vi "Localization.vi"(10 "parameter":string, 11 "Unlocalized":string="Launched") -> (3 "Localized":string="Launched TSS Server !")   [LabVIEW 2025, in "Config Tool.lvlib"]
doc: "This VI is used to provide localization -- that is, support for other human languages -- in the user interface. Given an input string, this VI returns the string that should be displayed for the current language. The idea is that you as a developer can use the Export/Import Strings feature of LabVIEW to produce a file that a translator can localize. The convention is that any control with \"DNL_\" as its label is skipped during localization (in English, this stands for Do Not Localize). The first array in this VI is one of these DNL_ controls. This array has the fixed strings that the program uses. The second array has the translated strings. Using this for all user visible text is sometimes cumbersome on the programmer, but it limits how many VIs have to be reviewed for localization.\n\nEven if you are not translating into other languages, this style of string lookup provides a central location for all your user visible text, which you may reuse at multiple points in your program, thus making it easy for tech writers to review for spelling or to make late-in-development-cycle changes with minimal risk to the rest of the code."
uses:
  Config Tool.lvlib
panel:
  in  "Localized Array":string[](array[string])=["Test Stand Software%s", "Initializing GUI...%s", "Reading %s...", "Opening %s...", "Loading User Interface, Please Wait...%s", "Initializing Plugin...%s", "Launched TSS Server !%s", "Done!%s", "TSS", "Current Action:"]
  in  "Unlocalized Array":string[](array[string])=["Splash Screen Title", "UI", "Read INI File", "Open File", "Loading Application", "PlugIn", "Launched", "Done!", "App Name", "Current Action:"]
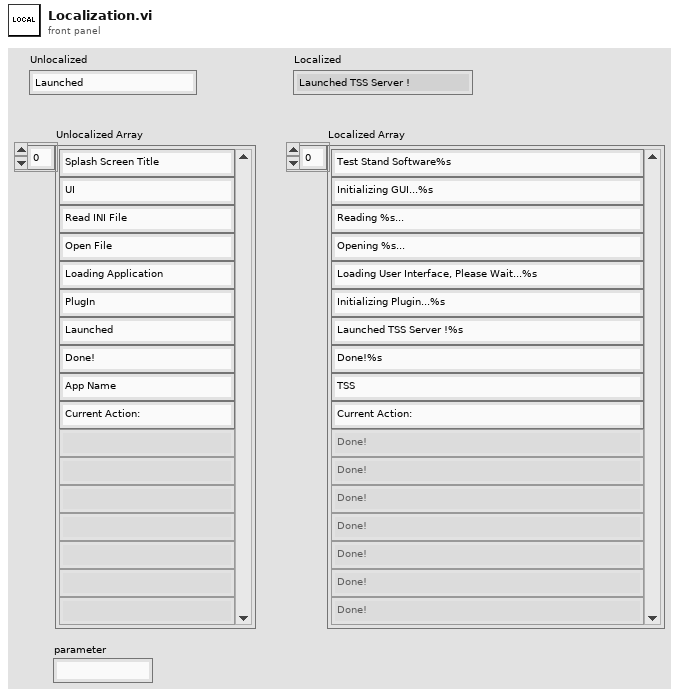
[diagram p1: front panel]
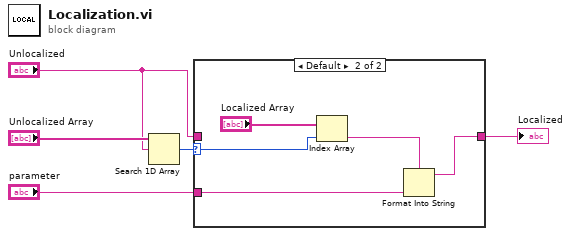
[diagram p0: block diagram]
diagram:
  n1 = Search 1D Array(1D array="Unlocalized Array", element="Unlocalized") -> (index of element=w3:i32)  [unwired: 1 in]
  n2 = case shown="Default" w3 {
    selector: w3 -> [_ w10]
    tunnel: [w6 w8] -> w4
    tunnel: "Unlocalized" -> [w6 _]
    tunnel: "parameter" -> [_ w7]
    frame ..-1 {
    }
    frame Default {
      n3 = Index Array(array="Localized Array", index=w10) -> (element=w9:string)
      n4 = Format Into String(format string=w9, w7) -> (resulting string=w8:string)  [unwired: 2 in, 1 out]
    }
  }
  "Localized" <- w4
